vi "Configure Trigger Select.vi"(4 "Hold Type (0: TI)":u16(ring) items=["TI", "PS", "PL", "PE", "IS", "IL", "IE"], 6 "Trigger type":u16(ring) items=["Edge", "Pulse", "Slope", "Video"], 7 "Trigger Source (1: Channel 1)":u16(ring)=1 items=["Channel 1"=1, "Channel 2"=2, "Channel 3"=3, "Channel 4"=4, "Ext"=5, "Ext5"=6, "AC Line"=7], 8 "error in (no error)":errorcluster, 10 "Hold Value (100 ns)":dbl=1e-07 format="%#_3g", 11 "VISA resource name":refnum<visa-resource-name>) -> (0 "error out":errorcluster, 3 "VISA resource name out":refnum<visa-resource-name>)   [LabVIEW 2021, in "Siglent SDS 1000 2000 Series.lvlib"]
doc: "Selects the condition that will trigger the acquisition of waveforms. Depending on the trigger type, additional parameters may need to be specified."
uses:
  <instrlib>/Siglent SDS 1000 2000 Series/Siglent SDS 1000 2000 Series.lvlib
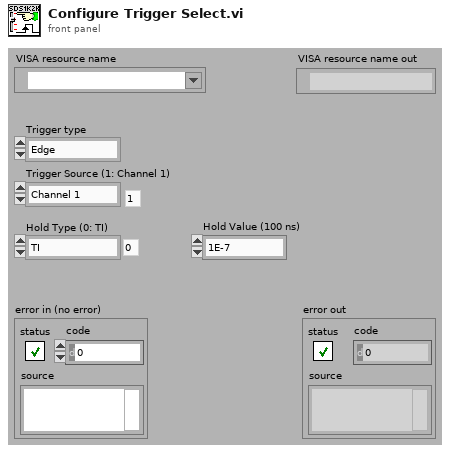
[diagram p1: front panel]
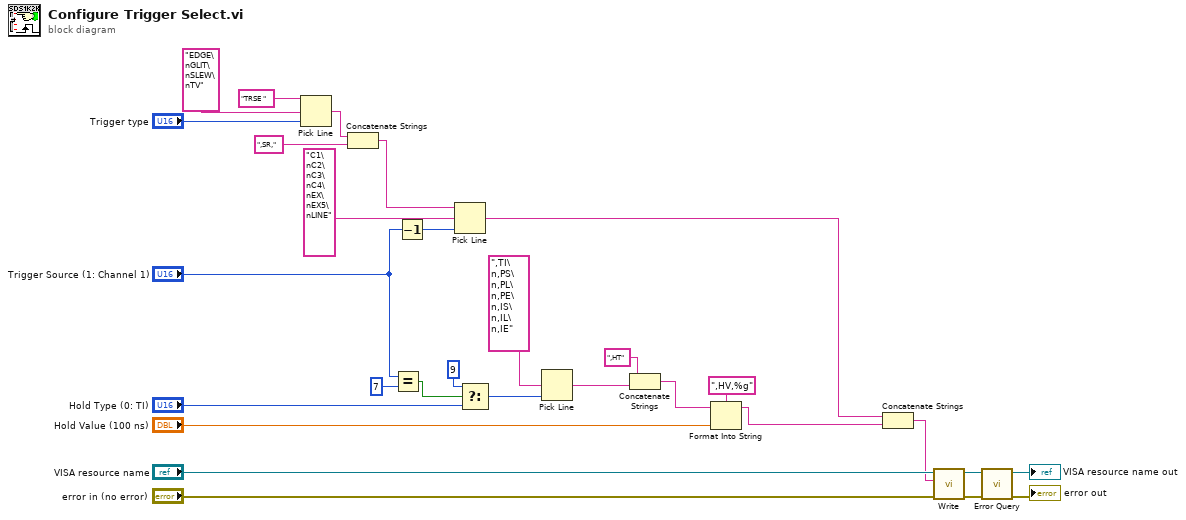
[diagram p0: block diagram]
diagram:
  n1 = Pick Line(string ("")="TRSE ", multi-line string="EDGE\nGLIT\nSLEW\nTV", line index="Trigger type") -> (output string=w21:string)
  n2 = Concatenate Strings(w21, ",SR,") -> (w22:string)
  n3 = Equal?(x="Trigger Source (1: Channel 1)", y=u16 7) -> (x = y?=w15:bool)
  n4 = Decrement(x="Trigger Source (1: Channel 1)") -> (x-1=w5:u16)
  n5 = Pick Line(string ("")=w22, multi-line string="C1\nC2\nC3\nC4\nEX\nEX5\nLINE", line index=w5) -> (output string=w6:string)
  n6 = Select(t=u16 9, s=w15, f="Hold Type (0: TI)") -> (s? t:f=w11:u16)
  n7 = Pick Line(multi-line string=",TI\n,PS\n,PL\n,PE\n,IS\n,IL\n,IE", line index=w11) -> (output string=w19:string)  [unwired: 1 in]
  n8 = Concatenate Strings(",HT", w19) -> (w1:string)
  n9 = Format Into String(format string=",HV,%g", initial string=w1, "Hold Value (100 ns)") -> (resulting string=w17:string)  [unwired: 1 in, 1 out]
  n10 = Concatenate Strings(w6, w17) -> (w16:string)
  n11 = call <instrlib>:"Write.vi"("error in (no error)"="error in (no error)", "Write Buffer"=w16, "VISA resource name"="VISA resource name") -> ("error out"=w9:errorcluster, "VISA resource name out"=w10:refnum<visa-resource-name>)  [unwired: 6 in, 1 out]
  n12 = call <instrlib>:"Error Query.vi"("error in (no error)"=w9, "VISA resource name"=w10) -> ("error out"=→"error out":errorcluster, "VISA resource name out"=→"VISA resource name out":refnum<visa-resource-name>)  [unwired: 6 in, 2 out]
